vi "Get Typedef Name.vi"(1 "Embedded Message Name":string, 2 "Generate_SerializationHelper":bool) -> (0 "To be nested\n message ctl":string)   [LabVIEW 2019, in "gRPC Template Creation Utility.lvlib"]
uses:
  gRPC Template Creation Utility.lvlib
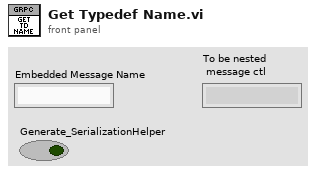
[diagram p1: front panel]
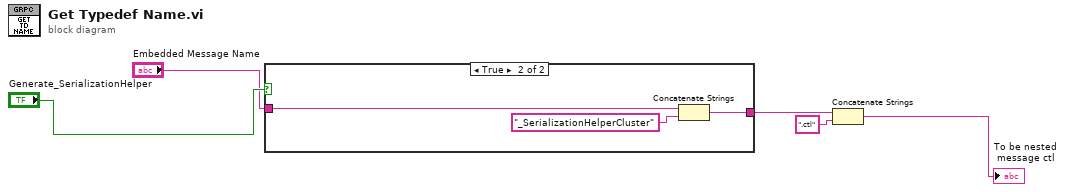
[diagram p0: block diagram]
diagram:
  n1 = case shown="True" "Generate_SerializationHelper" {
    tunnel: "Embedded Message Name" -> [w6 w9]
    tunnel: [w6 w8] -> w3
    frame False {
    }
    frame True {
      n2 = Concatenate Strings(w9, "_SerializationHelperCluster" ("string")) -> (w8:string)
    }
  }
  n3 = Concatenate Strings(w3, ".ctl" ("string")) -> (→"To be nested\n message ctl":string)
